vi "getOffset.vi"(8 "error in (no error)":errorcluster, 11 "IReaderStatus in":refnum<class "IReaderStatus.lvclass">) -> (0 "error out":errorcluster, 2 "Offset out":i64, 3 "IReaderStatus out":refnum<class "IReaderStatus.lvclass">)   [LabVIEW 2022 SP3, in "openDAQ.lvlib" / "IBaseObject.lvlib" / "IReaderStatus.lvlib" / "IReaderStatus.lvclass"]
uses:
  <instrlib>/openDAQ/Public/Classes/IReaderStatus/IReaderStatus.lvclass
  C:/Program Files (x86)/National Instruments/LabVIEW 2022/instr.lib/openDAQ/Public/Classes/IBaseObject/IBaseObject.lvclass
  <instrlib>/openDAQ/Public/Classes/daqCoreTypes/INumber/INumber.lvclass
  <instrlib>/openDAQ/Public/Classes/IBaseObject/IBaseObject.lvclass/IBaseObject.ctl
  <instrlib>/openDAQ/Public/Classes/IBaseObject/Accessor/Read reference.vi
  <instrlib>/openDAQ/Public/Classes/IBaseObject/Accessor/Write reference.vi
  <instrlib>/openDAQ/Binaries/Windows/x86/copendaq32.dll
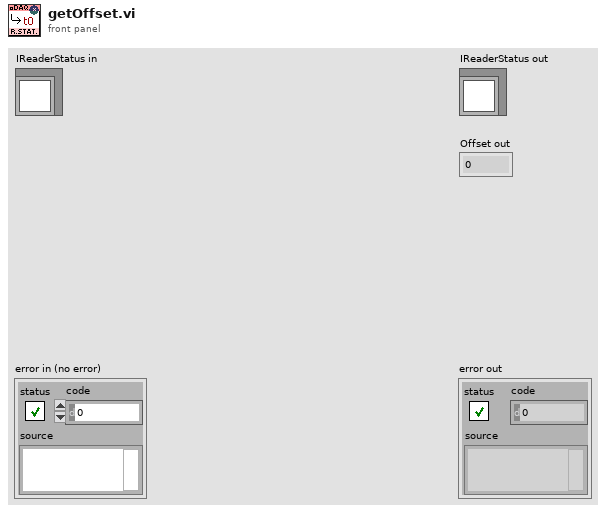
[diagram p1: front panel]
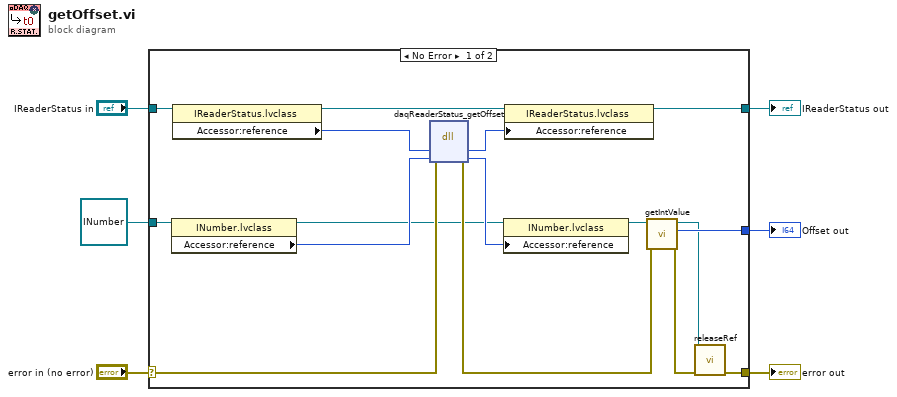
[diagram p0: block diagram]
diagram:
  n1 = case shown="No Error" "error in (no error)" {
    selector: "error in (no error)" -> [w18 w24]
    tunnel: [w9 w24] -> w5
    tunnel: [w16 w23] -> w3
    tunnel: "IReaderStatus in" -> [w19 w23]
    tunnel: refnum<class "INumber.lvclass"> refnum ("openDAQ.lvlib:daqCoreTypes.lvlib:INumber.lvclass") -> [w13 _]
    tunnel: [w20 _] -> w1
    frame No Error {
      n2 = property class="INumber.lvclass"(reference=w13) -> (reference out=w11:refnum<class "INumber.lvclass">, "Accessor:reference"=w12:i64)  [unwired: 1 in, 1 out]
      n3 = property class="IReaderStatus.lvclass"(reference=w19) -> (reference out=w17:refnum<class "IReaderStatus.lvclass">, "Accessor:reference"=w15:i64)  [unwired: 1 in, 1 out]
      n4 = dll-call lib="C:/Program Files (x86)/National Instruments/LabVIEW 2022/instr.lib/openDAQ/Binaries/Windows/x86/copendaq*.*" fn="daqReaderStatus_getOffset"(error in=w18, "readerStatus"=w15, "offset"=w12) -> (error out=w21:errorcluster, "readerStatus"=w14:i64, "offset"=w22:i64)  [unwired: 3 in, 1 out]
      n5 = property class="INumber.lvclass"(reference=w11, "Accessor:reference"=w22) -> (reference out=w10:refnum<class "INumber.lvclass">)  [unwired: 1 in, 1 out]
      n6 = property class="IReaderStatus.lvclass"(reference=w17, "Accessor:reference"=w14) -> (reference out=w16:refnum<class "IReaderStatus.lvclass">)  [unwired: 1 in, 1 out]
      n7 = call <instrlib>:"getIntValue.vi"("error in (no error)"=w21, "INumber in"=w10) -> ("error out"=w8:errorcluster, "Int Value out"=w20:i64, "INumber out"=w7:refnum<class "INumber.lvclass">)  [unwired: 7 in]
      n8 = call-dynamic "releaseRef.vi"("error in (no error)"=w8, "IBaseObject in"=w7) -> ("error out"=w9:errorcluster)  [unwired: 9 in]
    }
    frame Error {
    }
  }
  "error out" <- w5
  "IReaderStatus out" <- w3
  "Offset out" <- w1
